vi "proyecto.vi"() -> ()   [LabVIEW 2019]
uses:
  <vilib>/MakerHub/LINX/Public/Peripherals/Digital/Digital Write 1 Chan.vi
  <vilib>/MakerHub/LINX/Public/Peripherals/Analog/Analog Read 1 Chan.vi
  <vilib>/MakerHub/LINX/Public/Peripherals/PWM/PWM Set Duty Cycle 1 Chan.vi
  <vilib>/MakerHub/LINX/Public/Peripherals/Digital/Digital Write N Chans.vi
  <vilib>/MakerHub/LINX/Public/Peripherals/Analog/Analog Read N Chans.vi
  <vilib>/MakerHub/LINX/Private/Local IO/LinxDigitalWrite.vi
  <vilib>/MakerHub/LINX/Public/Utilities/Check Channel.vi
  <vilib>/MakerHub/LINX/Private/Local IO/LinxAnalogRead.vi
  <vilib>/MakerHub/LINX/Public/Utilities/Open Serial.vi
  <vilib>/MakerHub/LINX/Private/Utilties/Generate Error.vi
  <vilib>/MakerHub/LINX/Public/Peripherals/PWM/PWM Set Duty Cycle N Chans.vi
  <vilib>/MakerHub/LINX/LMH-LINX.lvlib
  <vilib>/Analysis/NI_AALPro.lvlib
panel:
  out "inf":dbl
  out "INf":string
  out "slope 3":dbl
  out "c3":string
  out "C2":string
  out "C1":string
  out "slope 2":dbl
  out "slope":dbl
  in  "Archivo C2":path
  out "Resultat final":string="No trobat"
  in  "Archivo C3":path
  in  "Archivo c1":path
  in  "Nombre plastico":string="Ambiente"
  in  "Archivo infrarojo":path
  in  "Accion":string(combo)="Medida C3"
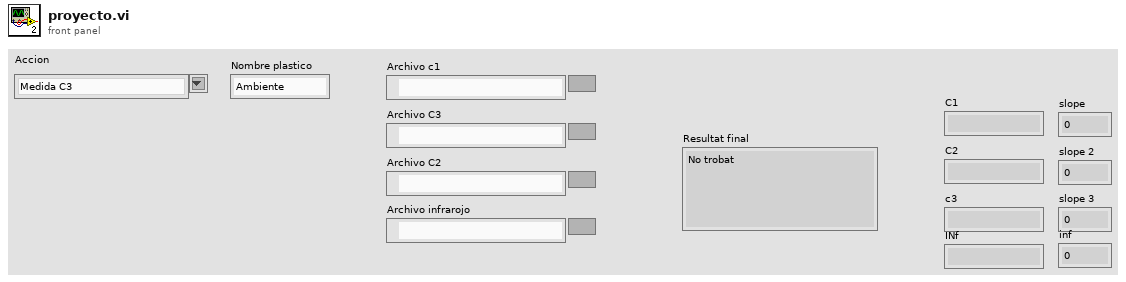
[diagram p1: front panel]
types:
  T1 = enum16{"open", "replace", "create", "open or create", "replace or create", "replace or create with confirmation"}
  T2 = typedef "LMH-LINX.lvlib/LINX Ref.ctl" = cluster{"IO":T3, "Interface":T4, "LINX Device Config":T5}
  T3 = typedef "LMH-LINX.lvlib/Platform.ctl" = enum16{"Remote", "Local"}
  T4 = typedef "LMH-LINX.lvlib/Interface.ctl" = enum16{"Serial", "TCP"}
  T5 = typedef "LMH-LINX.lvlib/Device.lvlib/LINX Device Config.ctl" = cluster{"Interface":T4, "COM Port":refnum<visa-resource-name>, "TCP Configuration":T6, "Device Family":u8, "Device ID":u8, "Device Name":string, "TCP Ref":refnum<k5>, "Channels":T7}
  T6 = typedef "LMH-LINX.lvlib/Device.lvlib/TCP Config.ctl" = cluster{"IP Address":string, "Port":u16}
  T7 = typedef "LMH-LINX.lvlib/Channels.ctl" = cluster{"DI":u8[], "DO":u8[], "AI":u8[], "AO":u8[], "PWM":u8[], "QE":u8[], "UART":u8[], "I2C 2":u8[], "SPI":u8[], "CAN":u8[], "Servo":u8[], "AI Ref (V)":dbl, "AI Resolution (Bits)":u8, "AO Ref (V)":dbl, "AO Resolution (Bits)":u8}
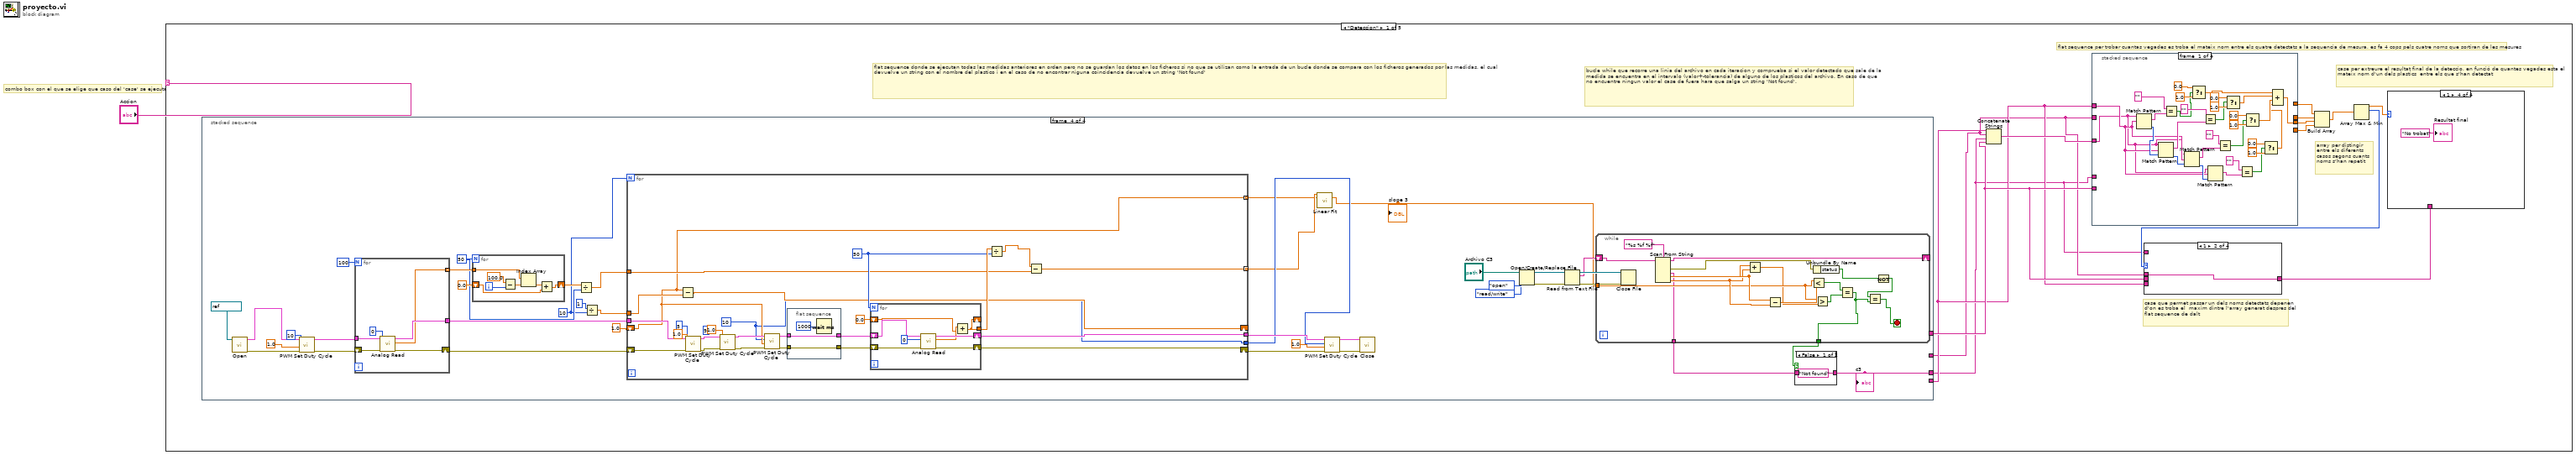
[diagram p0: block diagram]
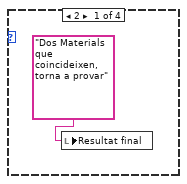
[diagram p5: hidden frame]
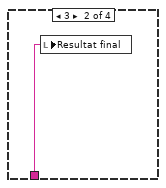
[diagram p6: hidden frame]
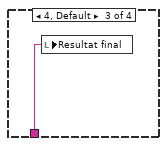
[diagram p7: hidden frame]
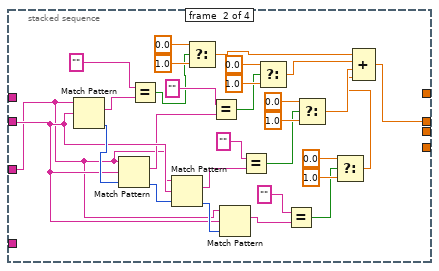
[diagram p8: hidden frame]
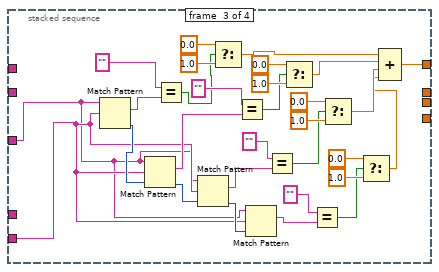
[diagram p9: hidden frame]
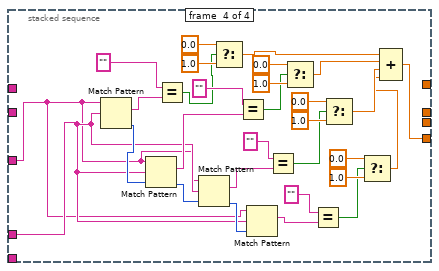
[diagram p10: hidden frame]
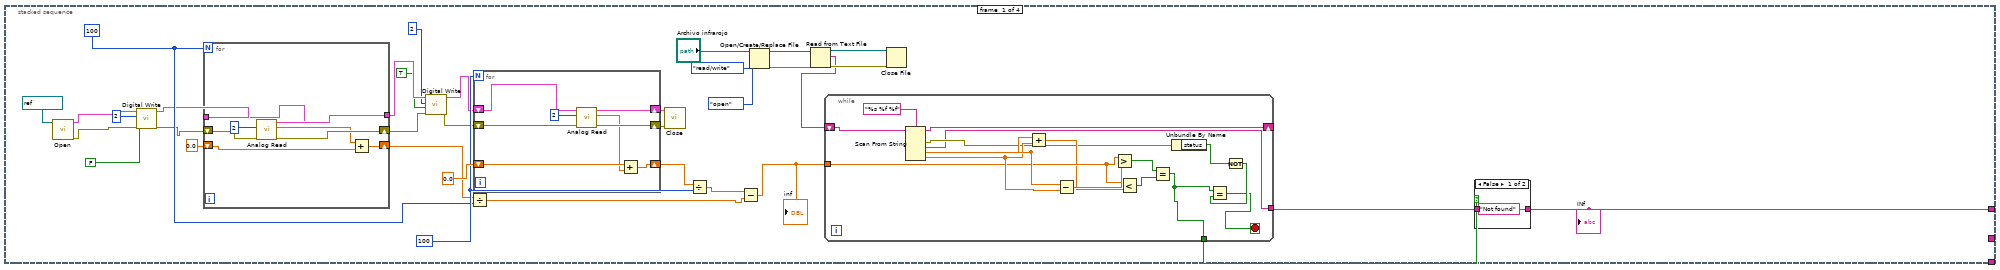
[diagram p11: hidden frame]
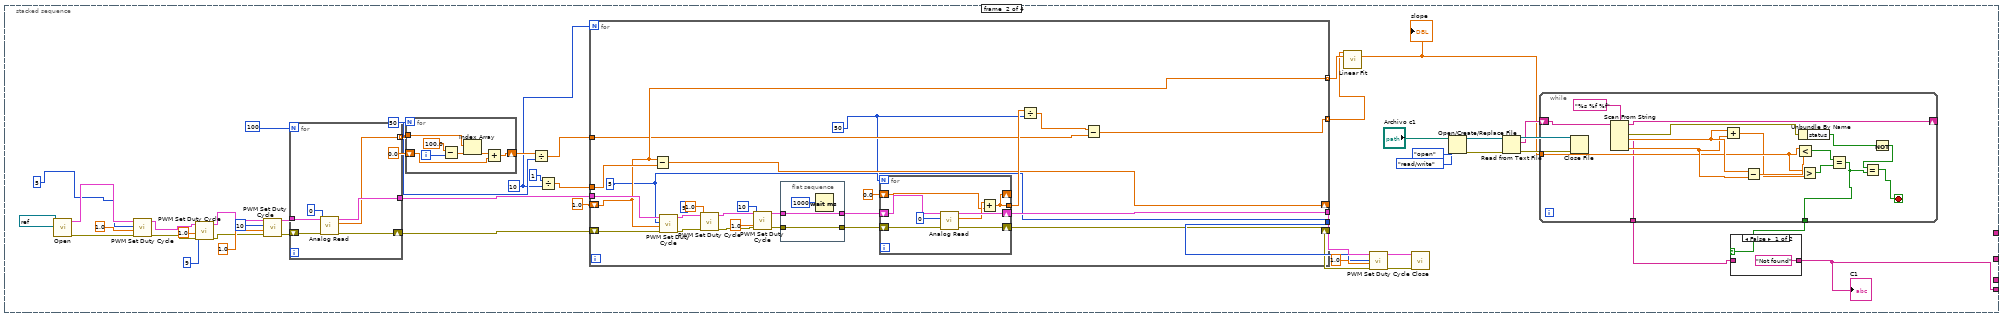
[diagram p13: hidden frame]
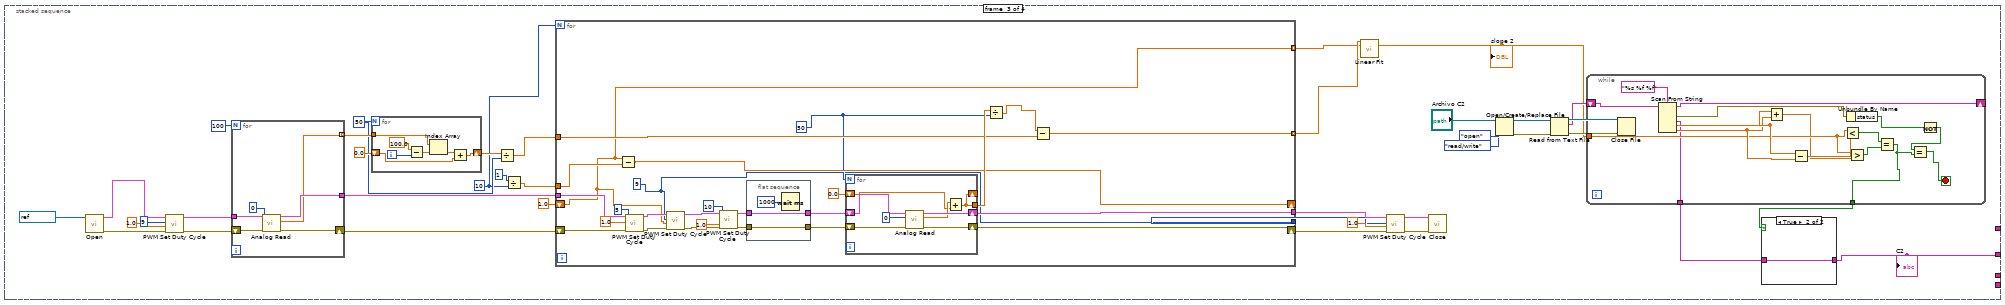
[diagram p15: hidden frame]
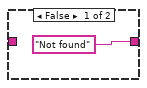
[diagram p16: hidden frame]
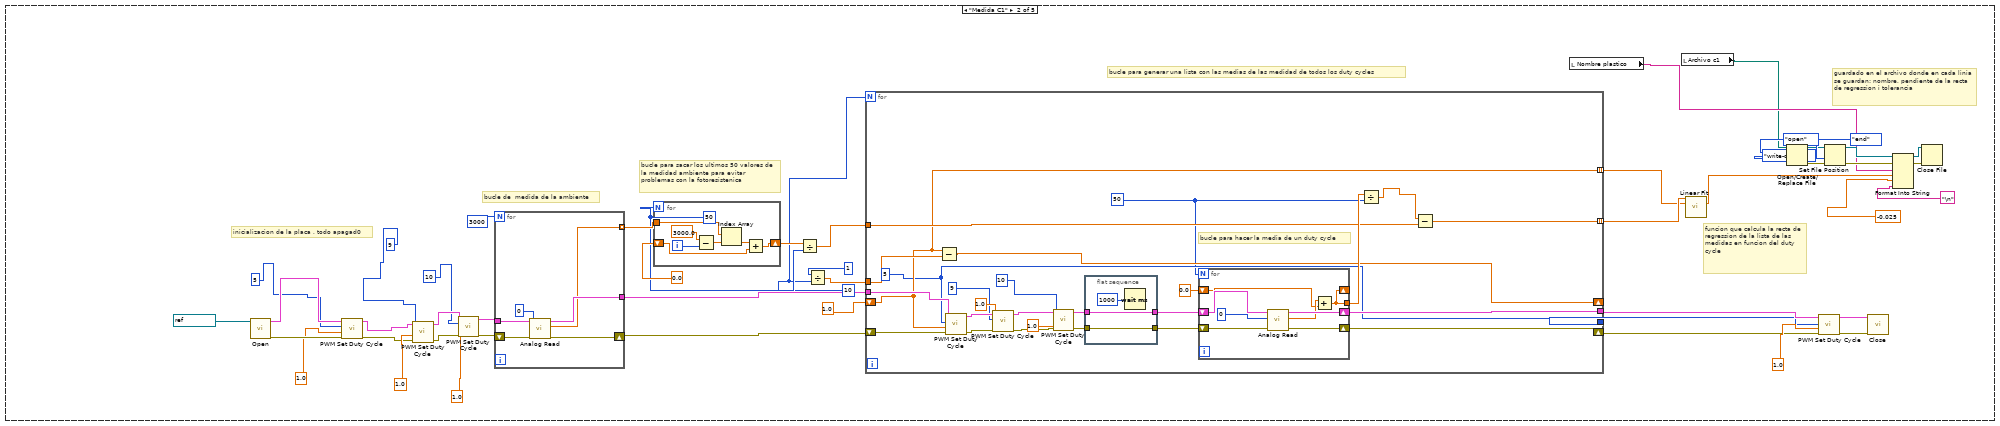
[diagram p18: hidden frame]
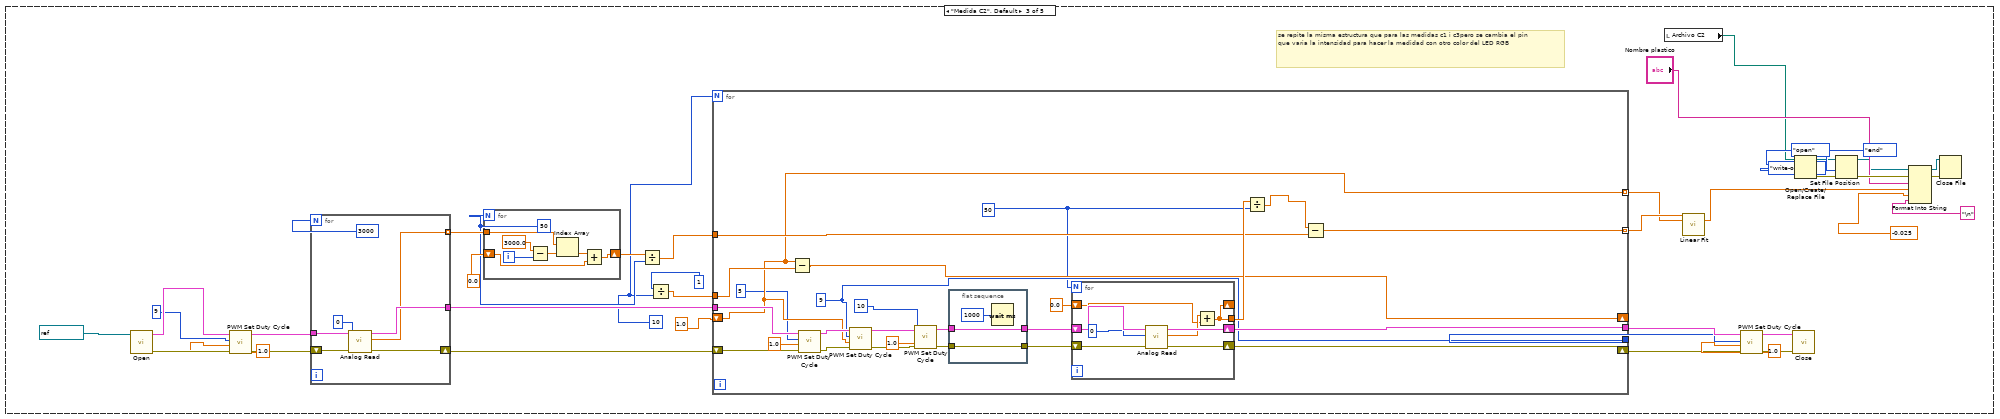
[diagram p19: hidden frame]
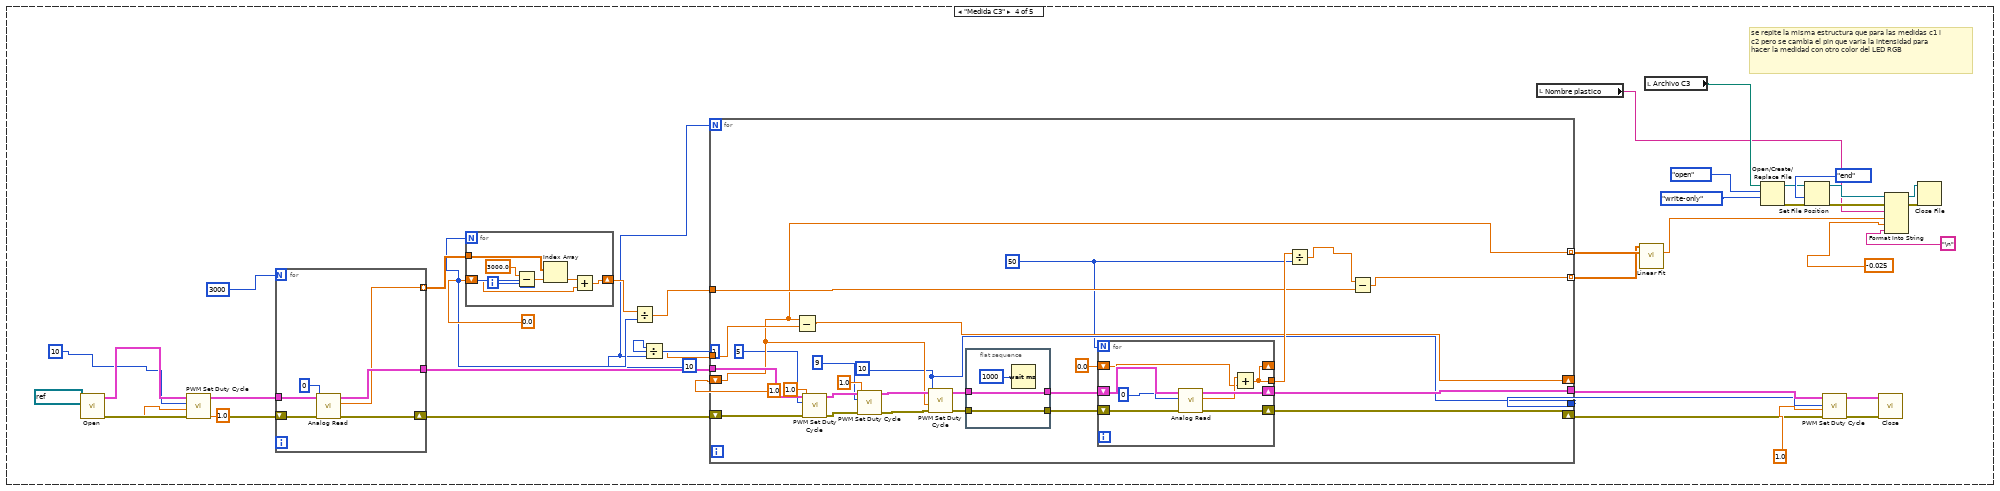
[diagram p20: hidden frame]
diagram:
  # "combo box con el que se elige que caso del 'case' se ejecuta"
  n1 = case shown="\"Deteccion\"" "Accion" {
    frame "Deteccion" {
      # "array per distingir entre els diferents casos segons cuants noms s'han repetit"
      # "case que permet passar un dels noms detectats depenen d'on es troba el  maxim dintre l'array generat despres del flat sequence de dalt"
      # "case per extreure el resultat final de la deteccio, en funció de quantes vegades esta el mateix nom d'un dels plastics  entre els que s'han detectat"
      # "flat sequence per trobar cuantas vegades es troba el mateix nom entre els quatre detectats a la sequencia de mesura, es fa 4 cops pels cuatre noms que sortiran de les mesures"
      # "bucle while que recorre una linia del archivo en cada iteracion y comprueba si el valor detectado que sale de la medida se encuentra en el intervalo (valor+-tolerancia) de alguno de los plasticos del archivo. En caso de que no encuentre ningun valor el case de fuera hara que salga un string 'Not found'."
      # "flat sequence donde se ejecutan todas las medidas anteriores en orden pero no se guardan los datos en los ficheros si no que se utilizan como la entrada de un bucle donde se compara con los ficheros generados por las medidas, el cual devuelve un string con el nombre del plastico i en el caso de no encontrar niguna coincidencia devuelve un string 'Not found'"
      n2 = stacked-sequence {
        tunnel: [_ w212 _ _] -> w4
        tunnel: [_ _ w333 _] -> w3
        tunnel: [_ _ _ w439] -> w2
        tunnel: [w147 _ _ _] -> w5
        frame #0 {
          w172 = 100 ("Numero de muestras 2")
          w170 = 100
          n3 = call-poly <vilib>:"Open.vi"("Serial Port"=refnum<visa-resource-name> "COM3") -> ("Error Out"=w168:errorcluster, "LINX Resource"=w169:T2)  [unwired: 8 in, 1 out]
          n4 = call-poly <vilib>:"Digital Write.vi"("Error In"=w168, "Output Value"=FALSE, "DO Channel"=u8 2, "LINX Resource"=w169) -> ("Error Out"=w166:errorcluster, "LINX Resource"=w165:T2)  [unwired: 6 in]
          n5 = for {
            N: w170 -> [_]
            tunnel: [w203] -> w164
            shift-right: [w202] -> w162
            shift-left: w166 -> [w199]
            shift-right: [w201] -> w171
            shift-left: 0.0 -> [w198]
            tunnel: w165 -> [w200]
            n6 = call-poly <vilib>:"Analog Read.vi"("Error In"=w199, "Analog Channel"=u8 2, "LINX Resource"=w200) -> ("Error Out"=w202:errorcluster, "Voltage"=w197:dbl, "LINX Resource"=w203:T2)  [unwired: 5 in, 1 out]
            n7 = Add(x=w197, y=w198) -> (x+y=w201:dbl)
          }
          n8 = call-poly <vilib>:"Digital Write.vi"("Error In"=w162, "Output Value"=TRUE, "DO Channel"=u8 2, "LINX Resource"=w164) -> ("Error Out"=w161:errorcluster, "LINX Resource"=w163:T2)  [unwired: 6 in]
          n9 = Divide(x=w171, y=w170) -> (x/y=w157:dbl)
          n10 = for {
            N: w172 -> [_]
            shift-right: [w210] -> w176
            shift-left: w163 -> [w211]
            shift-right: [w208] -> w175
            shift-left: w161 -> [w209]
            shift-right: [w206] -> w173
            shift-left: 0.0 -> [w207]
            n11 = call-poly <vilib>:"Analog Read.vi"("Error In"=w209, "Analog Channel"=u8 2, "LINX Resource"=w211) -> ("Error Out"=w208:errorcluster, "Voltage"=w205:dbl, "LINX Resource"=w210:T2)  [unwired: 5 in, 1 out]
            n12 = Add(x=w207, y=w205) -> (x+y=w206:dbl)
          }
          n13 = call <vilib>:"Close.vi"("Error In"=w175, "LINX Resource"=w176) -> ()  [unwired: 9 in, 1 out]
          n14 = Divide(x=w173, y=w172) -> (x/y=w158:dbl)
          n15 = Subtract(x=w158, y=w157) -> (x-y=w150:dbl)
          "inf" <- w150
          n16 = Open/Create/Replace File(file path (use dialog)="Archivo infrarojo", operation (0:open)=T1."open", access (0:read/write)=enum16{"read/write", "read-only", "write-only"}."read/write") -> (refnum out=w155:refnum<file>, error out=w153:errorcluster)  [unwired: 3 in, 1 out]
          n17 = Read from Text File(file (use dialog)=w155, error in=w153) -> (refnum out=w154:refnum<file>, text=w151:string, error out=w152:errorcluster)  [unwired: 2 in, 1 out]
          n18 = while {
            shift-right: [w195] -> _
            shift-left: w151 -> [w194]
            tunnel: w150 -> [w189]
            tunnel: [w183] -> w148
            tunnel: [w180] -> w149
            stop <- w181 stop-if-true
            n19 = Scan From String(format string="%s %f %f", input string=w194) -> (remaining string=w195:string, error out=w185:errorcluster, output 1=w180:string, output 2=w192:dbl, output 3=w191:dbl)  [unwired: 5 in, 1 out]
            n20 = Add(x=w192, y=w191) -> (x+y=w188:dbl)
            n21 = Subtract(x=w192, y=w191) -> (x-y=w190:dbl)
            n22 = Greater?(x=w189, y=w190) -> (0:w187:bool)
            n23 = Less?(x=w189, y=w188) -> (x < y?=w186:bool)
            n24 = Equal?(x=w187, y=w186) -> (x = y?=w183:bool)
            n25 = Unbundle By Name(w185) -> ("status"=w184:bool)
            n26 = Not(x=w184) -> (.not. x?=w182:bool)
            n27 = Equal?(x=w183, y=w182) -> (x = y?=w181:bool)
          }
          n28 = Close File(refnum=w154, error in=w152) -> ()  [unwired: 2 out]
          n29 = case shown="False" w148 {
            tunnel: ["Not found" w179] -> w147
            tunnel: w149 -> [_ w179]
            frame False {
            }
            frame True {
            }
          }
          "INf" <- w147
        }
        frame #1 {
          w241 = 50
          w238 = 10
          n30 = call-poly <vilib>:"Open.vi"("Serial Port"=refnum<visa-resource-name> "COM3") -> ("Error Out"=w246:errorcluster, "LINX Resource"=w247:T2)  [unwired: 8 in, 1 out]
          n31 = call-poly <vilib>:"PWM Set Duty Cycle.vi"("Error In"=w246, "Duty Cycle (0-1)"=1.0, "PWM Channel"=u8 5, "LINX Resource"=w247) -> ("Error Out"=w235:errorcluster, "LINX Resource"=w236:T2)  [unwired: 6 in]
          n32 = call-poly <vilib>:"PWM Set Duty Cycle.vi"("Error In"=w235, "Duty Cycle (0-1)"=1.0, "PWM Channel"=u8 9, "LINX Resource"=w236) -> ("Error Out"=w232:errorcluster, "LINX Resource"=w233:T2)  [unwired: 6 in]
          n33 = call-poly <vilib>:"PWM Set Duty Cycle.vi"("Error In"=w232, "Duty Cycle (0-1)"=1.0, "PWM Channel"=u8 10, "LINX Resource"=w233) -> ("Error Out"=w230:errorcluster, "LINX Resource"=w231:T2)  [unwired: 6 in]
          n34 = for {
            N: 100 -> [_]
            tunnel: [w289] -> w240
            shift-right: [w288] -> w239
            shift-left: w230 -> [w286]
            tunnel: w231 -> [w287]
            tunnel: [w285] -> w244 mode=indexing
            n35 = call-poly <vilib>:"Analog Read.vi"("Error In"=w286, "Analog Channel"=u8 0, "LINX Resource"=w287) -> ("Error Out"=w288:errorcluster, "Voltage"=w285:dbl, "LINX Resource"=w289:T2)  [unwired: 5 in, 1 out]
          }
          n36 = for {
            N: w241 -> [_]
            tunnel: w244 -> [w280]
            shift-right: [w277] -> w242
            shift-left: 0.0 -> [w279]
            i -> [w282]
            n37 = Subtract(x=100.0, y=w282) -> (x-y=w281:dbl)
            n38 = Index Array(array=w280, index=w281) -> (element=w278:dbl)
            n39 = Add(x=w278, y=w279) -> (x+y=w277:dbl)
          }
          n40 = Divide(x=w242, y=w241) -> (x/y=w248:dbl)
          n41 = Divide(x=1, y=w238) -> (x/y=w252:dbl)
          n42 = for {
            N: w238 -> [_]
            tunnel: w240 -> [w315]
            tunnel: [w314] -> w258
            tunnel: [w292] -> w254
            shift-right: [w306] -> _
            shift-left: 1.0 -> [w297]
            tunnel: w252 -> [w307]
            shift-right: [w308] -> w250
            shift-left: w239 -> [w309]
            tunnel: w248 -> [w295]
            tunnel: [w297] -> w229 mode=indexing
            tunnel: [w294] -> w228 mode=indexing
            w292 = u8 5 ("PWM Channel")
            w293 = 50
            n43 = Subtract(x=w297, y=w307) -> (x-y=w306:dbl)
            n44 = call-poly <vilib>:"PWM Set Duty Cycle.vi"("Error In"=w309, "Duty Cycle (0-1)"=w297, "PWM Channel"=w292, "LINX Resource"=w315) -> ("Error Out"=w304:errorcluster, "LINX Resource"=w305:T2)  [unwired: 6 in]
            n45 = call-poly <vilib>:"PWM Set Duty Cycle.vi"("Error In"=w304, "Duty Cycle (0-1)"=1.0, "PWM Channel"=u8 9, "LINX Resource"=w305) -> ("Error Out"=w300:errorcluster, "LINX Resource"=w301:T2)  [unwired: 6 in]
            n46 = call-poly <vilib>:"PWM Set Duty Cycle.vi"("Error In"=w300, "Duty Cycle (0-1)"=1.0, "PWM Channel"=u8 10, "LINX Resource"=w301) -> ("Error Out"=w299:errorcluster, "LINX Resource"=w298:T2)  [unwired: 6 in]
            n47 = flat-sequence {
              tunnel: [w326] -> w313
              tunnel: w298 -> [w326]
              tunnel: [w325] -> w312
              tunnel: w299 -> [w325]
              frame #0 {
                n48 = Wait (ms)(milliseconds to wait=u32 1000) -> ()  [unwired: 1 out]
              }
            }
            n49 = for {
              N: w293 -> [_]
              shift-right: [w323] -> w314
              shift-left: w313 -> [w321]
              shift-right: [w322] -> w308
              shift-left: w312 -> [w320]
              shift-right: [w317] -> _
              shift-left: 0.0 -> [w318]
              tunnel: [w317] -> w310
              n50 = call-poly <vilib>:"Analog Read.vi"("Error In"=w320, "Analog Channel"=u8 0, "LINX Resource"=w321) -> ("Error Out"=w322:errorcluster, "Voltage"=w319:dbl, "LINX Resource"=w323:T2)  [unwired: 5 in, 1 out]
              n51 = Add(x=w319, y=w318) -> (x+y=w317:dbl)
            }
            n52 = Divide(x=w310, y=w293) -> (x/y=w296:dbl)
            n53 = Subtract(x=w296, y=w295) -> (x-y=w294:dbl)
          }
          n54 = call <vilib>:"Linear Fit.vi"("Y"=w228, "X"=w229) -> ("slope"=w221:dbl)  [unwired: 9 in, 4 out]
          "slope" <- w221
          n55 = call-poly <vilib>:"PWM Set Duty Cycle.vi"("Error In"=w250, "Duty Cycle (0-1)"=1.0, "PWM Channel"=w254, "LINX Resource"=w258) -> ("Error Out"=w256:errorcluster, "LINX Resource"=w255:T2)  [unwired: 6 in]
          n56 = call <vilib>:"Close.vi"("Error In"=w256, "LINX Resource"=w255) -> ()  [unwired: 9 in, 1 out]
          n57 = Open/Create/Replace File(file path (use dialog)="Archivo c1", operation (0:open)=T1."open", access (0:read/write)=enum16{"read/write", "read-only", "write-only"}."read/write") -> (refnum out=w226:refnum<file>, error out=w224:errorcluster)  [unwired: 3 in, 1 out]
          n58 = Read from Text File(file (use dialog)=w226, error in=w224) -> (refnum out=w225:refnum<file>, text=w222:string, error out=w223:errorcluster)  [unwired: 2 in, 1 out]
          n59 = while {
            shift-right: [w276] -> _
            shift-left: w222 -> [w275]
            tunnel: w221 -> [w270]
            tunnel: [w263] -> w220
            tunnel: [w261] -> w219
            stop <- w262 stop-if-true
            n60 = Scan From String(format string="%s %f %f", input string=w275) -> (remaining string=w276:string, error out=w266:errorcluster, output 1=w261:string, output 2=w273:dbl, output 3=w272:dbl)  [unwired: 5 in, 1 out]
            n61 = Add(x=w273, y=w272) -> (x+y=w269:dbl)
            n62 = Subtract(x=w273, y=w272) -> (x-y=w271:dbl)
            n63 = Less?(x=w270, y=w271) -> (x < y?=w268:bool)
            n64 = Unbundle By Name(w266) -> ("status"=w265:bool)
            n65 = Greater?(x=w270, y=w269) -> (0:w267:bool)
            n66 = Equal?(x=w268, y=w267) -> (x = y?=w263:bool)
            n67 = Not(x=w265) -> (.not. x?=w264:bool)
            n68 = Equal?(x=w264, y=w263) -> (x = y?=w262:bool)
          }
          n69 = Close File(refnum=w225, error in=w223) -> ()  [unwired: 2 out]
          n70 = case shown="False" w220 {
            tunnel: ["Not found" w260] -> w212
            tunnel: w219 -> [_ w260]
            frame False {
            }
            frame True {
            }
          }
          "C1" <- w212
        }
        frame #2 {
          w346 = 50
          w343 = 10
          n71 = call-poly <vilib>:"Open.vi"("Serial Port"=refnum<visa-resource-name> "COM3" ("Serial Port 5")) -> ("Error Out"=w353:errorcluster, "LINX Resource"=w354:T2)  [unwired: 8 in, 1 out]
          n72 = call-poly <vilib>:"PWM Set Duty Cycle.vi"("Error In"=w353, "Duty Cycle (0-1)"=1.0, "PWM Channel"=u8 9, "LINX Resource"=w354) -> ("Error Out"=w350:errorcluster, "LINX Resource"=w351:T2)  [unwired: 6 in]
          n73 = for {
            N: 100 -> [_]
            tunnel: [w396] -> w345
            shift-right: [w395] -> w344
            shift-left: w350 -> [w393]
            tunnel: w351 -> [w394]
            tunnel: [w392] -> w349 mode=indexing
            n74 = call-poly <vilib>:"Analog Read.vi"("Error In"=w393, "Analog Channel"=u8 0, "LINX Resource"=w394) -> ("Error Out"=w395:errorcluster, "Voltage"=w392:dbl, "LINX Resource"=w396:T2)  [unwired: 5 in, 1 out]
          }
          n75 = for {
            N: w346 -> [_]
            tunnel: w349 -> [w387]
            shift-right: [w384] -> w347
            shift-left: 0.0 -> [w386]
            i -> [w389]
            n76 = Subtract(x=100.0, y=w389) -> (x-y=w388:dbl)
            n77 = Index Array(array=w387, index=w388) -> (element=w385:dbl)
            n78 = Add(x=w385, y=w386) -> (x+y=w384:dbl)
          }
          n79 = Divide(x=w347, y=w346) -> (x/y=w355:dbl)
          n80 = Divide(x=1, y=w343) -> (x/y=w359:dbl)
          n81 = for {
            N: w343 -> [_]
            tunnel: w345 -> [w422]
            tunnel: [w421] -> w365
            tunnel: [w398] -> w361
            shift-right: [w411] -> _
            shift-left: 1.0 -> [w401]
            tunnel: w359 -> [w412]
            shift-right: [w415] -> w357
            shift-left: w344 -> [w416]
            tunnel: w355 -> [w414]
            tunnel: [w402] -> w342 mode=indexing
            tunnel: [w401] -> w341 mode=indexing
            w398 = u8 9 ("PWM Channel")
            w400 = 50
            n82 = Subtract(x=w401, y=w412) -> (x-y=w411:dbl)
            n83 = call-poly <vilib>:"PWM Set Duty Cycle.vi"("Error In"=w416, "Duty Cycle (0-1)"=1.0, "PWM Channel"=u8 5, "LINX Resource"=w422) -> ("Error Out"=w409:errorcluster, "LINX Resource"=w410:T2)  [unwired: 6 in]
            n84 = call-poly <vilib>:"PWM Set Duty Cycle.vi"("Error In"=w409, "Duty Cycle (0-1)"=w401, "PWM Channel"=w398, "LINX Resource"=w410) -> ("Error Out"=w406:errorcluster, "LINX Resource"=w407:T2)  [unwired: 6 in]
            n85 = call-poly <vilib>:"PWM Set Duty Cycle.vi"("Error In"=w406, "Duty Cycle (0-1)"=1.0, "PWM Channel"=u8 10, "LINX Resource"=w407) -> ("Error Out"=w405:errorcluster, "LINX Resource"=w404:T2)  [unwired: 6 in]
            n86 = flat-sequence {
              tunnel: [w433] -> w420
              tunnel: w404 -> [w433]
              tunnel: [w432] -> w419
              tunnel: w405 -> [w432]
              frame #0 {
                n87 = Wait (ms)(milliseconds to wait=u32 1000) -> ()  [unwired: 1 out]
              }
            }
            n88 = for {
              N: w400 -> [_]
              shift-right: [w430] -> w421
              shift-left: w420 -> [w428]
              shift-right: [w429] -> w415
              shift-left: w419 -> [w427]
              shift-right: [w424] -> _
              shift-left: 0.0 -> [w425]
              tunnel: [w424] -> w417
              n89 = call-poly <vilib>:"Analog Read.vi"("Error In"=w427, "Analog Channel"=u8 0, "LINX Resource"=w428) -> ("Error Out"=w429:errorcluster, "Voltage"=w426:dbl, "LINX Resource"=w430:T2)  [unwired: 5 in, 1 out]
              n90 = Add(x=w426, y=w425) -> (x+y=w424:dbl)
            }
            n91 = Divide(x=w417, y=w400) -> (x/y=w413:dbl)
            n92 = Subtract(x=w413, y=w414) -> (x-y=w402:dbl)
          }
          n93 = call <vilib>:"Linear Fit.vi"("Y"=w342, "X"=w341) -> ("slope"=w335:dbl)  [unwired: 9 in, 4 out]
          "slope 2" <- w335
          n94 = call-poly <vilib>:"PWM Set Duty Cycle.vi"("Error In"=w357, "Duty Cycle (0-1)"=1.0, "PWM Channel"=w361, "LINX Resource"=w365) -> ("Error Out"=w363:errorcluster, "LINX Resource"=w362:T2)  [unwired: 6 in]
          n95 = call <vilib>:"Close.vi"("Error In"=w363, "LINX Resource"=w362) -> ()  [unwired: 9 in, 1 out]
          n96 = Open/Create/Replace File(file path (use dialog)="Archivo C2", operation (0:open)=T1."open", access (0:read/write)=enum16{"read/write", "read-only", "write-only"}."read/write") -> (refnum out=w340:refnum<file>, error out=w338:errorcluster)  [unwired: 3 in, 1 out]
          n97 = Read from Text File(file (use dialog)=w340, error in=w338) -> (refnum out=w339:refnum<file>, text=w336:string, error out=w337:errorcluster)  [unwired: 2 in, 1 out]
          n98 = while {
            shift-right: [w383] -> _
            shift-left: w336 -> [w382]
            tunnel: w335 -> [w377]
            tunnel: [w370] -> w334
            tunnel: [w368] -> w328
            stop <- w369 stop-if-true
            n99 = Scan From String(format string="%s %f %f", input string=w382) -> (remaining string=w383:string, error out=w373:errorcluster, output 1=w368:string, output 2=w380:dbl, output 3=w379:dbl)  [unwired: 5 in, 1 out]
            n100 = Add(x=w380, y=w379) -> (x+y=w376:dbl)
            n101 = Subtract(x=w380, y=w379) -> (x-y=w378:dbl)
            n102 = Less?(x=w377, y=w378) -> (x < y?=w375:bool)
            n103 = Unbundle By Name(w373) -> ("status"=w372:bool)
            n104 = Greater?(x=w377, y=w376) -> (0:w374:bool)
            n105 = Equal?(x=w375, y=w374) -> (x = y?=w370:bool)
            n106 = Not(x=w372) -> (.not. x?=w371:bool)
            n107 = Equal?(x=w371, y=w370) -> (x = y?=w369:bool)
          }
          n108 = Close File(refnum=w339, error in=w337) -> ()  [unwired: 2 out]
          n109 = case shown="True" w334 {
            tunnel: ["Not found" w367] -> w333
            tunnel: w328 -> [_ w367]
            frame False {
            }
            frame True {
            }
          }
          "C2" <- w333
        }
        frame #3 {
          w453 = 50
          w450 = 10
          n110 = call-poly <vilib>:"Open.vi"("Serial Port"=refnum<visa-resource-name> "COM3") -> ("Error Out"=w460:errorcluster, "LINX Resource"=w461:T2)  [unwired: 8 in, 1 out]
          n111 = call-poly <vilib>:"PWM Set Duty Cycle.vi"("Error In"=w460, "Duty Cycle (0-1)"=1.0, "PWM Channel"=u8 10, "LINX Resource"=w461) -> ("Error Out"=w457:errorcluster, "LINX Resource"=w458:T2)  [unwired: 6 in]
          n112 = for {
            N: 100 -> [_]
            tunnel: [w503] -> w452
            shift-right: [w502] -> w451
            shift-left: w457 -> [w500]
            tunnel: w458 -> [w501]
            tunnel: [w499] -> w456 mode=indexing
            n113 = call-poly <vilib>:"Analog Read.vi"("Error In"=w500, "Analog Channel"=u8 0, "LINX Resource"=w501) -> ("Error Out"=w502:errorcluster, "Voltage"=w499:dbl, "LINX Resource"=w503:T2)  [unwired: 5 in, 1 out]
          }
          n114 = for {
            N: w453 -> [_]
            tunnel: w456 -> [w494]
            shift-right: [w491] -> w454
            shift-left: 0.0 -> [w493]
            i -> [w496]
            n115 = Subtract(x=100.0, y=w496) -> (x-y=w495:dbl)
            n116 = Index Array(array=w494, index=w495) -> (element=w492:dbl)
            n117 = Add(x=w492, y=w493) -> (x+y=w491:dbl)
          }
          n118 = Divide(x=w454, y=w453) -> (x/y=w462:dbl)
          n119 = Divide(x=1, y=w450) -> (x/y=w466:dbl)
          n120 = for {
            N: w450 -> [_]
            tunnel: w452 -> [w529]
            tunnel: [w528] -> w472
            tunnel: [w504] -> w468
            shift-right: [w517] -> _
            shift-left: 1.0 -> [w507]
            tunnel: w466 -> [w518]
            shift-right: [w521] -> w464
            shift-left: w451 -> [w522]
            tunnel: w462 -> [w520]
            tunnel: [w508] -> w449 mode=indexing
            tunnel: [w507] -> w448 mode=indexing
            w504 = u8 10 ("PWM Channel")
            w523 = 50 ("Numero de punts per cada duty 6")
            n121 = Subtract(x=w507, y=w518) -> (x-y=w517:dbl)
            n122 = call-poly <vilib>:"PWM Set Duty Cycle.vi"("Error In"=w522, "Duty Cycle (0-1)"=1.0, "PWM Channel"=u8 5, "LINX Resource"=w529) -> ("Error Out"=w515:errorcluster, "LINX Resource"=w516:T2)  [unwired: 6 in]
            n123 = call-poly <vilib>:"PWM Set Duty Cycle.vi"("Error In"=w515, "Duty Cycle (0-1)"=1.0, "PWM Channel"=u8 9, "LINX Resource"=w516) -> ("Error Out"=w512:errorcluster, "LINX Resource"=w513:T2)  [unwired: 6 in]
            n124 = call-poly <vilib>:"PWM Set Duty Cycle.vi"("Error In"=w512, "Duty Cycle (0-1)"=w507, "PWM Channel"=w504, "LINX Resource"=w513) -> ("Error Out"=w511:errorcluster, "LINX Resource"=w510:T2)  [unwired: 6 in]
            n125 = flat-sequence {
              tunnel: [w540] -> w527
              tunnel: w510 -> [w540]
              tunnel: [w539] -> w526
              tunnel: w511 -> [w539]
              frame #0 {
                n126 = Wait (ms)(milliseconds to wait=u32 1000) -> ()  [unwired: 1 out]
              }
            }
            n127 = for {
              N: w523 -> [_]
              shift-right: [w537] -> w528
              shift-left: w527 -> [w535]
              shift-right: [w536] -> w521
              shift-left: w526 -> [w534]
              shift-right: [w531] -> _
              shift-left: 0.0 -> [w532]
              tunnel: [w531] -> w524
              n128 = call-poly <vilib>:"Analog Read.vi"("Error In"=w534, "Analog Channel"=u8 0, "LINX Resource"=w535) -> ("Error Out"=w536:errorcluster, "Voltage"=w533:dbl, "LINX Resource"=w537:T2)  [unwired: 5 in, 1 out]
              n129 = Add(x=w533, y=w532) -> (x+y=w531:dbl)
            }
            n130 = Divide(x=w524, y=w523) -> (x/y=w519:dbl)
            n131 = Subtract(x=w519, y=w520) -> (x-y=w508:dbl)
          }
          n132 = call <vilib>:"Linear Fit.vi"("Y"=w449, "X"=w448) -> ("slope"=w441:dbl)  [unwired: 9 in, 4 out]
          "slope 3" <- w441
          n133 = call-poly <vilib>:"PWM Set Duty Cycle.vi"("Error In"=w464, "Duty Cycle (0-1)"=1.0, "PWM Channel"=w468, "LINX Resource"=w472) -> ("Error Out"=w470:errorcluster, "LINX Resource"=w469:T2)  [unwired: 6 in]
          n134 = call <vilib>:"Close.vi"("Error In"=w470, "LINX Resource"=w469) -> ()  [unwired: 9 in, 1 out]
          n135 = Open/Create/Replace File(file path (use dialog)="Archivo C3", operation (0:open)=T1."open", access (0:read/write)=enum16{"read/write", "read-only", "write-only"}."read/write") -> (refnum out=w446:refnum<file>, error out=w444:errorcluster)  [unwired: 3 in, 1 out]
          n136 = Read from Text File(file (use dialog)=w446, error in=w444) -> (refnum out=w445:refnum<file>, text=w442:string, error out=w443:errorcluster)  [unwired: 2 in, 1 out]
          n137 = while {
            shift-right: [w490] -> _
            shift-left: w442 -> [w489]
            tunnel: w441 -> [w484]
            tunnel: [w477] -> w435
            tunnel: [w475] -> w440
            stop <- w476 stop-if-true
            n138 = Scan From String(format string="%s %f %f", input string=w489) -> (remaining string=w490:string, error out=w480:errorcluster, output 1=w475:string, output 2=w487:dbl, output 3=w486:dbl)  [unwired: 5 in, 1 out]
            n139 = Add(x=w487, y=w486) -> (x+y=w483:dbl)
            n140 = Subtract(x=w487, y=w486) -> (x-y=w485:dbl)
            n141 = Less?(x=w484, y=w485) -> (x < y?=w482:bool)
            n142 = Unbundle By Name(w480) -> ("status"=w479:bool)
            n143 = Greater?(x=w484, y=w483) -> (0:w481:bool)
            n144 = Equal?(x=w482, y=w481) -> (x = y?=w477:bool)
            n145 = Not(x=w479) -> (.not. x?=w478:bool)
            n146 = Equal?(x=w478, y=w477) -> (x = y?=w476:bool)
          }
          n147 = Close File(refnum=w445, error in=w443) -> ()  [unwired: 2 out]
          n148 = case shown="False" w435 {
            tunnel: ["Not found" w474] -> w439
            tunnel: w440 -> [_ w474]
            frame False {
            }
            frame True {
            }
          }
          "c3" <- w439
        }
      }
      n149 = Concatenate Strings(w4, w3, w2, w5) -> (w14:string)
      n150 = stacked-sequence {
        tunnel: w14 -> [w23 w53 w83 w113]
        tunnel: w4 -> [w25 _ _ _]
        tunnel: w3 -> [_ w79 _ _]
        tunnel: w2 -> [_ _ _ w115]
        tunnel: w5 -> [_ _ w85 _]
        tunnel: [_ _ w84 _] -> w13
        tunnel: [_ w54 _ _] -> w12
        tunnel: [w24 _ _ _] -> w11
        tunnel: [_ _ _ w114] -> w10
        frame #0 {
          n151 = Match Pattern(string=w23, regular expression=w25) -> (match substring=w48:string, offset past match=w52:i32)  [unwired: 1 in, 2 out]
          n152 = Match Pattern(string=w23, regular expression=w25, offset (0)=w52) -> (match substring=w44:string, offset past match=w51:i32)  [unwired: 2 out]
          n153 = Equal?(x="", y=w48) -> (x = y?=w33:bool)
          n154 = Match Pattern(string=w23, regular expression=w25, offset (0)=w51) -> (match substring=w43:string, offset past match=w50:i32)  [unwired: 2 out]
          n155 = Select(t=0.0, s=w33, f=1.0) -> (s? t:f=w29:dbl)
          n156 = Equal?(x="", y=w44) -> (x = y?=w32:bool)
          n157 = Match Pattern(string=w23, regular expression=w25, offset (0)=w50) -> (match substring=w42:string)  [unwired: 3 out]
          n158 = Equal?(x="", y=w43) -> (x = y?=w31:bool)
          n159 = Select(t=0.0, s=w32, f=1.0) -> (s? t:f=w28:dbl)
          n160 = Equal?(x="", y=w42) -> (x = y?=w30:bool)
          n161 = Select(t=0.0, s=w31, f=1.0) -> (s? t:f=w27:dbl)
          n162 = Select(t=0.0, s=w30, f=1.0) -> (s? t:f=w26:dbl)
          n163 = Compound Arithmetic op=ADD(w29, w28, w27, w26) -> (w24:dbl)
        }
        frame #1 {
          n164 = Match Pattern(string=w53, regular expression=w79) -> (match substring=w77:string, offset past match=w82:i32)  [unwired: 1 in, 2 out]
          n165 = Match Pattern(string=w53, regular expression=w79, offset (0)=w82) -> (match substring=w73:string, offset past match=w81:i32)  [unwired: 2 out]
          n166 = Equal?(x="", y=w77) -> (x = y?=w62:bool)
          n167 = Match Pattern(string=w53, regular expression=w79, offset (0)=w81) -> (match substring=w72:string, offset past match=w80:i32)  [unwired: 2 out]
          n168 = Select(t=0.0, s=w62, f=1.0) -> (s? t:f=w58:dbl)
          n169 = Equal?(x="", y=w73) -> (x = y?=w61:bool)
          n170 = Match Pattern(string=w53, regular expression=w79, offset (0)=w80) -> (match substring=w71:string)  [unwired: 3 out]
          n171 = Equal?(x="", y=w72) -> (x = y?=w60:bool)
          n172 = Select(t=0.0, s=w61, f=1.0) -> (s? t:f=w57:dbl)
          n173 = Equal?(x="", y=w71) -> (x = y?=w59:bool)
          n174 = Select(t=0.0, s=w60, f=1.0) -> (s? t:f=w56:dbl)
          n175 = Select(t=0.0, s=w59, f=1.0) -> (s? t:f=w55:dbl)
          n176 = Compound Arithmetic op=ADD(w58, w57, w56, w55) -> (w54:dbl)
        }
        frame #2 {
          n177 = Match Pattern(string=w83, regular expression=w85) -> (match substring=w108:string, offset past match=w112:i32)  [unwired: 1 in, 2 out]
          n178 = Match Pattern(string=w83, regular expression=w85, offset (0)=w112) -> (match substring=w104:string, offset past match=w111:i32)  [unwired: 2 out]
          n179 = Equal?(x="", y=w108) -> (x = y?=w93:bool)
          n180 = Match Pattern(string=w83, regular expression=w85, offset (0)=w111) -> (match substring=w103:string, offset past match=w110:i32)  [unwired: 2 out]
          n181 = Select(t=0.0, s=w93, f=1.0) -> (s? t:f=w89:dbl)
          n182 = Equal?(x="", y=w104) -> (x = y?=w92:bool)
          n183 = Match Pattern(string=w83, regular expression=w85, offset (0)=w110) -> (match substring=w102:string)  [unwired: 3 out]
          n184 = Equal?(x="", y=w103) -> (x = y?=w91:bool)
          n185 = Select(t=0.0, s=w92, f=1.0) -> (s? t:f=w88:dbl)
          n186 = Equal?(x="", y=w102) -> (x = y?=w90:bool)
          n187 = Select(t=0.0, s=w91, f=1.0) -> (s? t:f=w87:dbl)
          n188 = Select(t=0.0, s=w90, f=1.0) -> (s? t:f=w86:dbl)
          n189 = Compound Arithmetic op=ADD(w89, w88, w87, w86) -> (w84:dbl)
        }
        frame #3 {
          n190 = Match Pattern(string=w113, regular expression=w115) -> (match substring=w138:string, offset past match=w142:i32)  [unwired: 1 in, 2 out]
          n191 = Match Pattern(string=w113, regular expression=w115, offset (0)=w142) -> (match substring=w134:string, offset past match=w141:i32)  [unwired: 2 out]
          n192 = Equal?(x="", y=w138) -> (x = y?=w123:bool)
          n193 = Match Pattern(string=w113, regular expression=w115, offset (0)=w141) -> (match substring=w133:string, offset past match=w140:i32)  [unwired: 2 out]
          n194 = Select(t=0.0, s=w123, f=1.0) -> (s? t:f=w119:dbl)
          n195 = Equal?(x="", y=w134) -> (x = y?=w122:bool)
          n196 = Match Pattern(string=w113, regular expression=w115, offset (0)=w140) -> (match substring=w132:string)  [unwired: 3 out]
          n197 = Equal?(x="", y=w133) -> (x = y?=w121:bool)
          n198 = Select(t=0.0, s=w122, f=1.0) -> (s? t:f=w118:dbl)
          n199 = Equal?(x="", y=w132) -> (x = y?=w120:bool)
          n200 = Select(t=0.0, s=w121, f=1.0) -> (s? t:f=w117:dbl)
          n201 = Select(t=0.0, s=w120, f=1.0) -> (s? t:f=w116:dbl)
          n202 = Compound Arithmetic op=ADD(w119, w118, w117, w116) -> (w114:dbl)
        }
      }
      n203 = Build Array(w13, w12, w11, w10) -> (w9:dbl[])
      n204 = Array Max & Min(array=w9) -> (max value=w8:dbl, max index (indices)=w7:i32)  [unwired: 2 out]
      n205 = case shown="1" w7 {
        tunnel: [w15 w16 w17 w18] -> w6
        tunnel: w5 -> [w15 _ _ _]
        tunnel: w4 -> [_ _ w17 _]
        tunnel: w3 -> [_ w16 _ _]
        tunnel: w2 -> [_ _ _ w18]
        frame 0, Default {
        }
        frame 1 {
        }
        frame 2 {
        }
        frame 3 {
        }
      }
      n206 = case shown="1" w8 {
        tunnel: w6 -> [_ w20 w21 _]
        frame 2 {
          n207 = local write "Resultat final"("Dos Materials que coincideixen, torna a provar") -> ()
        }
        frame 3 {
          n208 = local write "Resultat final"(w20) -> ()
        }
        frame 4, Default {
          n209 = local write "Resultat final"(w21) -> ()
        }
        frame 1 {
          "Resultat final" <- "No trobat"
        }
      }
    }
    frame "Medida C1" {
      w572 = 50
      w569 = 10
      # "guardado en el archivo donde en cada linia se guardan: nombre, pendiente de la recta de regression i tolerancia"
      # "funcion que calcula la recta de regression de la lista de las medidas en funcion del duty cycle"
      # "bucle para generar una lista con las medias de las medidad de todos los duty cycles"
      # "bucle para sacar los ultimos 50 valores de la medidad ambiente para evitar problemas con la fotoresistenica"
      # "bucle de  medida de la ambiente"
      # "inicializacion de la placa , todo apagad0"
      n210 = call-poly <vilib>:"Open.vi"("Serial Port"=refnum<visa-resource-name> "COM3") -> ("Error Out"=w577:errorcluster, "LINX Resource"=w578:T2)  [unwired: 8 in, 1 out]
      n211 = call-poly <vilib>:"PWM Set Duty Cycle.vi"("Error In"=w577, "Duty Cycle (0-1)"=1.0, "PWM Channel"=u8 5, "LINX Resource"=w578) -> ("Error Out"=w566:errorcluster, "LINX Resource"=w567:T2)  [unwired: 6 in]
      n212 = call-poly <vilib>:"PWM Set Duty Cycle.vi"("Error In"=w566, "Duty Cycle (0-1)"=1.0, "PWM Channel"=u8 9, "LINX Resource"=w567) -> ("Error Out"=w563:errorcluster, "LINX Resource"=w564:T2)  [unwired: 6 in]
      n213 = call-poly <vilib>:"PWM Set Duty Cycle.vi"("Error In"=w563, "Duty Cycle (0-1)"=1.0, "PWM Channel"=u8 10, "LINX Resource"=w564) -> ("Error Out"=w561:errorcluster, "LINX Resource"=w562:T2)  [unwired: 6 in]
      n214 = for {
        N: 3000 -> [_]
        tunnel: [w602] -> w571
        shift-right: [w601] -> w570
        shift-left: w561 -> [w599]
        tunnel: w562 -> [w600]
        tunnel: [w598] -> w575 mode=indexing
        n215 = call-poly <vilib>:"Analog Read.vi"("Error In"=w599, "Analog Channel"=u8 0, "LINX Resource"=w600) -> ("Error Out"=w601:errorcluster, "Voltage"=w598:dbl, "LINX Resource"=w602:T2)  [unwired: 5 in, 1 out]
      }
      n216 = for {
        N: w572 -> [_]
        tunnel: w575 -> [w593]
        shift-right: [w590] -> w573
        shift-left: 0.0 -> [w592]
        i -> [w595]
        n217 = Subtract(x=3000.0, y=w595) -> (x-y=w594:dbl)
        n218 = Index Array(array=w593, index=w594) -> (element=w591:dbl)
        n219 = Add(x=w591, y=w592) -> (x+y=w590:dbl)
      }
      n220 = Divide(x=w573, y=w572) -> (x/y=w579:dbl)
      n221 = Divide(x=1, y=w569) -> (x/y=w583:dbl)
      n222 = for {
        N: w569 -> [_]
        tunnel: w571 -> [w628]
        tunnel: [w627] -> w589
        tunnel: [w606] -> w585
        shift-right: [w617] -> _
        shift-left: 1.0 -> [w607]
        tunnel: w583 -> [w618]
        shift-right: [w621] -> w581
        shift-left: w570 -> [w622]
        tunnel: w579 -> [w620]
        tunnel: [w608] -> w548 mode=indexing
        tunnel: [w607] -> w547 mode=indexing
        w603 = 50
        w606 = u8 5 ("PWM Channel")
        # "bucle para hacer la media de un duty cycle"
        n223 = Subtract(x=w607, y=w618) -> (x-y=w617:dbl)
        n224 = call-poly <vilib>:"PWM Set Duty Cycle.vi"("Error In"=w622, "Duty Cycle (0-1)"=w607, "PWM Channel"=w606, "LINX Resource"=w628) -> ("Error Out"=w615:errorcluster, "LINX Resource"=w616:T2)  [unwired: 6 in]
        n225 = call-poly <vilib>:"PWM Set Duty Cycle.vi"("Error In"=w615, "Duty Cycle (0-1)"=1.0, "PWM Channel"=u8 9, "LINX Resource"=w616) -> ("Error Out"=w611:errorcluster, "LINX Resource"=w612:T2)  [unwired: 6 in]
        n226 = call-poly <vilib>:"PWM Set Duty Cycle.vi"("Error In"=w611, "Duty Cycle (0-1)"=1.0, "PWM Channel"=u8 10, "LINX Resource"=w612) -> ("Error Out"=w610:errorcluster, "LINX Resource"=w609:T2)  [unwired: 6 in]
        n227 = flat-sequence {
          tunnel: [w639] -> w626
          tunnel: w609 -> [w639]
          tunnel: [w638] -> w625
          tunnel: w610 -> [w638]
          frame #0 {
            n228 = Wait (ms)(milliseconds to wait=u32 1000) -> ()  [unwired: 1 out]
          }
        }
        n229 = for {
          N: w603 -> [_]
          shift-right: [w636] -> w627
          shift-left: w626 -> [w634]
          shift-right: [w635] -> w621
          shift-left: w625 -> [w633]
          shift-right: [w630] -> _
          shift-left: 0.0 -> [w631]
          tunnel: [w630] -> w623
          n230 = call-poly <vilib>:"Analog Read.vi"("Error In"=w633, "Analog Channel"=u8 0, "LINX Resource"=w634) -> ("Error Out"=w635:errorcluster, "Voltage"=w632:dbl, "LINX Resource"=w636:T2)  [unwired: 5 in, 1 out]
          n231 = Add(x=w632, y=w631) -> (x+y=w630:dbl)
        }
        n232 = Divide(x=w623, y=w603) -> (x/y=w619:dbl)
        n233 = Subtract(x=w619, y=w620) -> (x-y=w608:dbl)
      }
      n234 = local read "Nombre plastico"() -> (w543:string)
      n235 = local read "Archivo c1"() -> (w542:path)
      n236 = call <vilib>:"Linear Fit.vi"("Y"=w548, "X"=w547) -> ("slope"=w549:dbl)  [unwired: 9 in, 4 out]
      n237 = Open/Create/Replace File(file path (use dialog)=w542, operation (0:open)=T1."open", access (0:read/write)=enum16{"read/write", "read-only", "write-only"}."write-only") -> (refnum out=w557:refnum<file>, error out=w556:errorcluster)  [unwired: 3 in, 1 out]
      n238 = call-poly <vilib>:"PWM Set Duty Cycle.vi"("Error In"=w581, "Duty Cycle (0-1)"=1.0, "PWM Channel"=w585, "LINX Resource"=w589) -> ("Error Out"=w587:errorcluster, "LINX Resource"=w586:T2)  [unwired: 6 in]
      n239 = Set File Position(refnum=w557, from (0:start)=enum16{"start", "end", "current"}."end", error in=w556) -> (refnum out=w551:refnum<file>, error out=w555:errorcluster)  [unwired: 1 in]
      n240 = call <vilib>:"Close.vi"("Error In"=w587, "LINX Resource"=w586) -> ()  [unwired: 9 in, 1 out]
      n241 = Format Into String(initial string=w551, error in=w555, w543, w549, -0.025 ("input 3"), "\n" ("input 4")) -> (resulting string=w554:refnum<file>, error out=w553:errorcluster)  [unwired: 1 in]
      n242 = Close File(refnum=w554, error in=w553) -> ()  [unwired: 2 out]
    }
    frame "Medida C2", Default {
      w662 = 50
      w659 = 10
      # "se repite la misma estructura que para las medidas c1 i c3pero se cambia el pin que varia la intensidad para hacer la medidad con otro color del LED RGB"
      n243 = call-poly <vilib>:"Open.vi"("Serial Port"=refnum<visa-resource-name> "COM3") -> ("Error Out"=w669:errorcluster, "LINX Resource"=w670:T2)  [unwired: 8 in, 1 out]
      n244 = call-poly <vilib>:"PWM Set Duty Cycle.vi"("Error In"=w669, "Duty Cycle (0-1)"=1.0, "PWM Channel"=u8 9, "LINX Resource"=w670) -> ("Error Out"=w666:errorcluster, "LINX Resource"=w667:T2)  [unwired: 6 in]
      n245 = for {
        N: 3000 -> [_]
        tunnel: [w693] -> w661
        shift-right: [w692] -> w660
        shift-left: w666 -> [w690]
        tunnel: w667 -> [w691]
        tunnel: [w689] -> w665 mode=indexing
        n246 = call-poly <vilib>:"Analog Read.vi"("Error In"=w690, "Analog Channel"=u8 0, "LINX Resource"=w691) -> ("Error Out"=w692:errorcluster, "Voltage"=w689:dbl, "LINX Resource"=w693:T2)  [unwired: 5 in, 1 out]
      }
      n247 = for {
        N: w662 -> [_]
        tunnel: w665 -> [w684]
        shift-right: [w681] -> w663
        shift-left: 0.0 -> [w683]
        i -> [w686]
        n248 = Subtract(x=3000.0, y=w686) -> (x-y=w685:dbl)
        n249 = Index Array(array=w684, index=w685) -> (element=w682:dbl)
        n250 = Add(x=w682, y=w683) -> (x+y=w681:dbl)
      }
      n251 = Divide(x=w663, y=w662) -> (x/y=w671:dbl)
      n252 = Divide(x=1, y=w659) -> (x/y=w675:dbl)
      n253 = for {
        N: w659 -> [_]
        tunnel: w661 -> [w719]
        tunnel: [w718] -> w680
        tunnel: [w696] -> w676
        shift-right: [w708] -> _
        shift-left: 1.0 -> [w698]
        tunnel: w675 -> [w709]
        shift-right: [w712] -> w673
        shift-left: w660 -> [w713]
        tunnel: w671 -> [w711]
        tunnel: [w699] -> w645 mode=indexing
        tunnel: [w698] -> w644 mode=indexing
        w694 = 50
        w696 = u8 9 ("PWM Channel")
        n254 = Subtract(x=w698, y=w709) -> (x-y=w708:dbl)
        n255 = call-poly <vilib>:"PWM Set Duty Cycle.vi"("Error In"=w713, "Duty Cycle (0-1)"=1.0, "PWM Channel"=u8 5, "LINX Resource"=w719) -> ("Error Out"=w706:errorcluster, "LINX Resource"=w707:T2)  [unwired: 6 in]
        n256 = call-poly <vilib>:"PWM Set Duty Cycle.vi"("Error In"=w706, "Duty Cycle (0-1)"=w698, "PWM Channel"=w696, "LINX Resource"=w707) -> ("Error Out"=w703:errorcluster, "LINX Resource"=w704:T2)  [unwired: 6 in]
        n257 = call-poly <vilib>:"PWM Set Duty Cycle.vi"("Error In"=w703, "Duty Cycle (0-1)"=1.0, "PWM Channel"=u8 10, "LINX Resource"=w704) -> ("Error Out"=w702:errorcluster, "LINX Resource"=w701:T2)  [unwired: 6 in]
        n258 = flat-sequence {
          tunnel: [w730] -> w717
          tunnel: w701 -> [w730]
          tunnel: [w729] -> w716
          tunnel: w702 -> [w729]
          frame #0 {
            n259 = Wait (ms)(milliseconds to wait=u32 1000) -> ()  [unwired: 1 out]
          }
        }
        n260 = for {
          N: w694 -> [_]
          shift-right: [w727] -> w718
          shift-left: w717 -> [w725]
          shift-right: [w726] -> w712
          shift-left: w716 -> [w724]
          shift-right: [w721] -> _
          shift-left: 0.0 -> [w722]
          tunnel: [w721] -> w714
          n261 = call-poly <vilib>:"Analog Read.vi"("Error In"=w724, "Analog Channel"=u8 0, "LINX Resource"=w725) -> ("Error Out"=w726:errorcluster, "Voltage"=w723:dbl, "LINX Resource"=w727:T2)  [unwired: 5 in, 1 out]
          n262 = Add(x=w723, y=w722) -> (x+y=w721:dbl)
        }
        n263 = Divide(x=w714, y=w694) -> (x/y=w710:dbl)
        n264 = Subtract(x=w710, y=w711) -> (x-y=w699:dbl)
      }
      n265 = local read "Archivo C2"() -> (w640:path)
      n266 = call <vilib>:"Linear Fit.vi"("Y"=w645, "X"=w644) -> ("slope"=w646:dbl)  [unwired: 9 in, 4 out]
      n267 = call-poly <vilib>:"PWM Set Duty Cycle.vi"("Error In"=w673, "Duty Cycle (0-1)"=1.0, "PWM Channel"=w676, "LINX Resource"=w680) -> ("Error Out"=w678:errorcluster, "LINX Resource"=w677:T2)  [unwired: 6 in]
      n268 = call <vilib>:"Close.vi"("Error In"=w678, "LINX Resource"=w677) -> ()  [unwired: 9 in, 1 out]
      n269 = Open/Create/Replace File(file path (use dialog)=w640, operation (0:open)=T1."open", access (0:read/write)=enum16{"read/write", "read-only", "write-only"}."write-only") -> (refnum out=w655:refnum<file>, error out=w654:errorcluster)  [unwired: 3 in, 1 out]
      n270 = Set File Position(refnum=w655, from (0:start)=enum16{"start", "end", "current"}."end", error in=w654) -> (refnum out=w648:refnum<file>, error out=w653:errorcluster)  [unwired: 1 in]
      n271 = Format Into String(initial string=w648, error in=w653, "Nombre plastico", w646, -0.025 ("input 3"), "\n" ("input 4")) -> (resulting string=w652:refnum<file>, error out=w651:errorcluster)  [unwired: 1 in]
      n272 = Close File(refnum=w652, error in=w651) -> ()  [unwired: 2 out]
    }
    frame "Medida C3" {
      w752 = 50
      w749 = 10
      # "se repite la misma estructura que para las medidas c1 i c2 pero se cambia el pin que varia la intensidad para hacer la medidad con otro color del LED RGB"
      n273 = call-poly <vilib>:"Open.vi"("Serial Port"=refnum<visa-resource-name> "COM3") -> ("Error Out"=w759:errorcluster, "LINX Resource"=w760:T2)  [unwired: 8 in, 1 out]
      n274 = call-poly <vilib>:"PWM Set Duty Cycle.vi"("Error In"=w759, "Duty Cycle (0-1)"=1.0, "PWM Channel"=u8 10, "LINX Resource"=w760) -> ("Error Out"=w756:errorcluster, "LINX Resource"=w757:T2)  [unwired: 6 in]
      n275 = for {
        N: 3000 -> [_]
        tunnel: [w784] -> w751
        shift-right: [w783] -> w750
        shift-left: w756 -> [w781]
        tunnel: w757 -> [w782]
        tunnel: [w780] -> w755 mode=indexing
        n276 = call-poly <vilib>:"Analog Read.vi"("Error In"=w781, "Analog Channel"=u8 0, "LINX Resource"=w782) -> ("Error Out"=w783:errorcluster, "Voltage"=w780:dbl, "LINX Resource"=w784:T2)  [unwired: 5 in, 1 out]
      }
      n277 = for {
        N: w752 -> [_]
        tunnel: w755 -> [w775]
        shift-right: [w772] -> w753
        shift-left: 0.0 -> [w774]
        i -> [w777]
        n278 = Subtract(x=3000.0, y=w777) -> (x-y=w776:dbl)
        n279 = Index Array(array=w775, index=w776) -> (element=w773:dbl)
        n280 = Add(x=w773, y=w774) -> (x+y=w772:dbl)
      }
      n281 = Divide(x=w753, y=w752) -> (x/y=w761:dbl)
      n282 = Divide(x=1, y=w749) -> (x/y=w765:dbl)
      n283 = for {
        N: w749 -> [_]
        tunnel: w751 -> [w810]
        tunnel: [w809] -> w771
        tunnel: [w786] -> w767
        shift-right: [w799] -> _
        shift-left: 1.0 -> [w790]
        tunnel: w765 -> [w800]
        shift-right: [w803] -> w763
        shift-left: w750 -> [w804]
        tunnel: w761 -> [w802]
        tunnel: [w790] -> w737 mode=indexing
        tunnel: [w789] -> w736 mode=indexing
        w785 = 50
        w786 = u8 10 ("PWM Channel")
        n284 = Subtract(x=w790, y=w800) -> (x-y=w799:dbl)
        n285 = call-poly <vilib>:"PWM Set Duty Cycle.vi"("Error In"=w804, "Duty Cycle (0-1)"=1.0, "PWM Channel"=u8 5, "LINX Resource"=w810) -> ("Error Out"=w797:errorcluster, "LINX Resource"=w798:T2)  [unwired: 6 in]
        n286 = call-poly <vilib>:"PWM Set Duty Cycle.vi"("Error In"=w797, "Duty Cycle (0-1)"=1.0, "PWM Channel"=u8 9, "LINX Resource"=w798) -> ("Error Out"=w794:errorcluster, "LINX Resource"=w795:T2)  [unwired: 6 in]
        n287 = call-poly <vilib>:"PWM Set Duty Cycle.vi"("Error In"=w794, "Duty Cycle (0-1)"=w790, "PWM Channel"=w786, "LINX Resource"=w795) -> ("Error Out"=w793:errorcluster, "LINX Resource"=w792:T2)  [unwired: 6 in]
        n288 = flat-sequence {
          tunnel: [w821] -> w808
          tunnel: w792 -> [w821]
          tunnel: [w820] -> w807
          tunnel: w793 -> [w820]
          frame #0 {
            n289 = Wait (ms)(milliseconds to wait=u32 1000) -> ()  [unwired: 1 out]
          }
        }
        n290 = for {
          N: w785 -> [_]
          shift-right: [w818] -> w809
          shift-left: w808 -> [w816]
          shift-right: [w817] -> w803
          shift-left: w807 -> [w815]
          shift-right: [w812] -> _
          shift-left: 0.0 -> [w813]
          tunnel: [w812] -> w805
          n291 = call-poly <vilib>:"Analog Read.vi"("Error In"=w815, "Analog Channel"=u8 0, "LINX Resource"=w816) -> ("Error Out"=w817:errorcluster, "Voltage"=w814:dbl, "LINX Resource"=w818:T2)  [unwired: 5 in, 1 out]
          n292 = Add(x=w814, y=w813) -> (x+y=w812:dbl)
        }
        n293 = Divide(x=w805, y=w785) -> (x/y=w801:dbl)
        n294 = Subtract(x=w801, y=w802) -> (x-y=w789:dbl)
      }
      n295 = local read "Nombre plastico"() -> (w731:string)
      n296 = call <vilib>:"Linear Fit.vi"("Y"=w736, "X"=w737) -> ("slope"=w735:dbl)  [unwired: 9 in, 4 out]
      n297 = local read "Archivo C3"() -> (w732:path)
      n298 = Open/Create/Replace File(file path (use dialog)=w732, operation (0:open)=T1."open", access (0:read/write)=enum16{"read/write", "read-only", "write-only"}."write-only") -> (refnum out=w745:refnum<file>, error out=w744:errorcluster)  [unwired: 3 in, 1 out]
      n299 = Set File Position(refnum=w745, from (0:start)=enum16{"start", "end", "current"}."end", error in=w744) -> (refnum out=w739:refnum<file>, error out=w743:errorcluster)  [unwired: 1 in]
      n300 = call-poly <vilib>:"PWM Set Duty Cycle.vi"("Error In"=w763, "Duty Cycle (0-1)"=1.0, "PWM Channel"=w767, "LINX Resource"=w771) -> ("Error Out"=w769:errorcluster, "LINX Resource"=w768:T2)  [unwired: 6 in]
      n301 = call <vilib>:"Close.vi"("Error In"=w769, "LINX Resource"=w768) -> ()  [unwired: 9 in, 1 out]
      n302 = Format Into String(initial string=w739, error in=w743, w731, w735, -0.025 ("input 3"), "\n" ("input 4")) -> (resulting string=w742:refnum<file>, error out=w741:errorcluster)  [unwired: 1 in]
      n303 = Close File(refnum=w742, error in=w741) -> ()  [unwired: 2 out]
    }
    frame "Medida infrarojo" {
      w827 = 500
      w839 = 100
      # "tolerancia"
      # "guardado de los datos en el fichero donde se guarda el nombre, el valor de la medidad, la tolerancia i una separacion para que la siguiente medidad se realice en la proxima linia"
      # "resta de la medidad hecha al ambiente a la media que sale del bucle"
      # "bucle de medida que devuelve la media de todas las medidas hechas"
      # "encendido del emisor para realizar la medidad"
      # "bucle de para hacer el analisis del ambiente donde el emisor esta apagado"
      # "inicazion del arduino: assignacion de pins i de inputs al circuito"
      n304 = call-poly <vilib>:"Open.vi"("Serial Port"=refnum<visa-resource-name> "COM3") -> ("Error Out"=w837:errorcluster, "LINX Resource"=w838:T2)  [unwired: 8 in, 1 out]
      n305 = call-poly <vilib>:"Digital Write.vi"("Error In"=w837, "Output Value"=FALSE, "DO Channel"=u8 2, "LINX Resource"=w838) -> ("Error Out"=w835:errorcluster, "LINX Resource"=w824:T2)  [unwired: 6 in]
      n306 = for {
        N: w839 -> [_]
        tunnel: [w866] -> w834
        shift-right: [w865] -> w832
        shift-left: w835 -> [w863]
        shift-right: [w864] -> w843
        shift-left: 0.0 -> [w862]
        tunnel: w824 -> [w860]
        n307 = call-poly <vilib>:"Analog Read.vi"("Error In"=w863, "Analog Channel"=u8 2, "LINX Resource"=w860) -> ("Error Out"=w865:errorcluster, "Voltage"=w859:dbl, "LINX Resource"=w866:T2)  [unwired: 5 in, 1 out]
        n308 = Add(x=w859, y=w862) -> (x+y=w864:dbl)
      }
      n309 = call-poly <vilib>:"Digital Write.vi"("Error In"=w832, "Output Value"=TRUE, "DO Channel"=u8 2 ("Analog Channel"), "LINX Resource"=w834) -> ("Error Out"=w831:errorcluster, "LINX Resource"=w833:T2)  [unwired: 6 in]
      n310 = Divide(x=w843, y=w839) -> (x/y=w841:dbl)
      n311 = for {
        N: w827 -> [_]
        shift-right: [w873] -> w857
        shift-left: w833 -> [w874]
        shift-right: [w871] -> w856
        shift-left: w831 -> [w872]
        shift-right: [w869] -> w854
        shift-left: 0.0 -> [w870]
        n312 = call-poly <vilib>:"Analog Read.vi"("Error In"=w872, "Analog Channel"=u8 2, "LINX Resource"=w874) -> ("Error Out"=w871:errorcluster, "Voltage"=w867:dbl, "LINX Resource"=w873:T2)  [unwired: 5 in, 1 out]
        n313 = Add(x=w870, y=w867) -> (x+y=w869:dbl)
      }
      n314 = local read "Nombre plastico"() -> (w822:string)
      n315 = call <vilib>:"Close.vi"("Error In"=w856, "LINX Resource"=w857) -> ()  [unwired: 9 in, 1 out]
      n316 = Divide(x=w854, y=w827) -> (x/y=w842:dbl)
      n317 = Subtract(x=w842, y=w841) -> (x-y=w840:dbl)
      n318 = local read "Archivo infrarojo"() -> (w823:path)
      n319 = Open/Create/Replace File(file path (use dialog)=w823, operation (0:open)=T1."open or create", access (0:read/write)=enum16{"read/write", "read-only", "write-only"}."write-only") -> (refnum out=w848:refnum<file>, error out=w849:errorcluster)  [unwired: 3 in, 1 out]
      n320 = Set File Position(refnum=w848, from (0:start)=enum16{"start", "end", "current"}."end", error in=w849) -> (refnum out=w847:refnum<file>, error out=w850:errorcluster)  [unwired: 1 in]
      n321 = Format Into String(initial string=w847, error in=w850, w822, w840, 0.005 ("input 3"), "\n" ("input 4")) -> (resulting string=w851:refnum<file>, error out=w852:errorcluster)  [unwired: 1 in]
      n322 = Close File(refnum=w851, error in=w852) -> ()  [unwired: 2 out]
    }
  }
